vi "170131-Counter - Continuous Output.vi"(8 "error in":errorcluster, 10 "Frequency":dbl=30.0 format="%.6f") -> (0 "error out 2":errorcluster={"status"=TRUE, "code"=-200220, "source"="DAQmx Create Channel (CO-Pulse Generation-Frequency).vi:4680002<append>\n<B>Device Specified: </B>Dev1\n<B>Suggested Device(s): </B>Dev4\n\n<B>Task Name: </B>_unnamedTask<4>"})   [LabVIEW 2017]
doc: "This example demonstrates how to continuously generate digital pulses using a counter output."
uses:
  <vilib>/DAQmx/create/channels.llb/DAQmx Create Channel (CO-Pulse Generation-Frequency).vi
  <vilib>/DAQmx/configure/timing.llb/DAQmx Timing (Implicit).vi
  <vilib>/DAQmx/configure/trigger.llb/DAQmx Start Trigger (Digital Edge).vi
  Global_InitEndSync.vi
  <resource>/objmgr/daqmx.rc
  <vilib>/Utility/error.llb/DialogType.ctl
panel:
  out "Actual Duty Cycle":dbl
  out "Actual Frequency":dbl
  in  "Duty Cycle":dbl=0.5 format="%.6f"
  in  "Output Terminal":tag="/PXI1Slot2/PFI24"
  in  "Trigger Type":T1(tab)
  in  "Edge":i32(ring)=10280 items=["Rising"=10280, "Falling"=10171]
  in  "Digital Trigger Source":tag
  in  "Pause When":i32(ring)=10192 items=["High"=10192, "Low"=10214]
  in  "Pause Trigger Source":tag
  in  "Stop":bool
  in  "Counter":tag="PXI1Slot2/ctr3"
  # "Channel Settings"
  # "Trigger Settings"
  # "To configure and use a trigger you must have the necessary tab selected above."
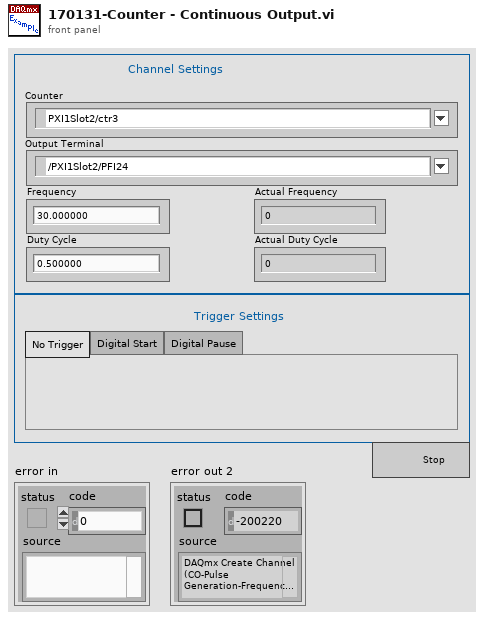
[diagram p1: front panel]
types:
  T1 = enum32{"No Trigger", "Digital Start", "Digital Pause"}
  T2 = typedef "DialogType.ctl" = u16
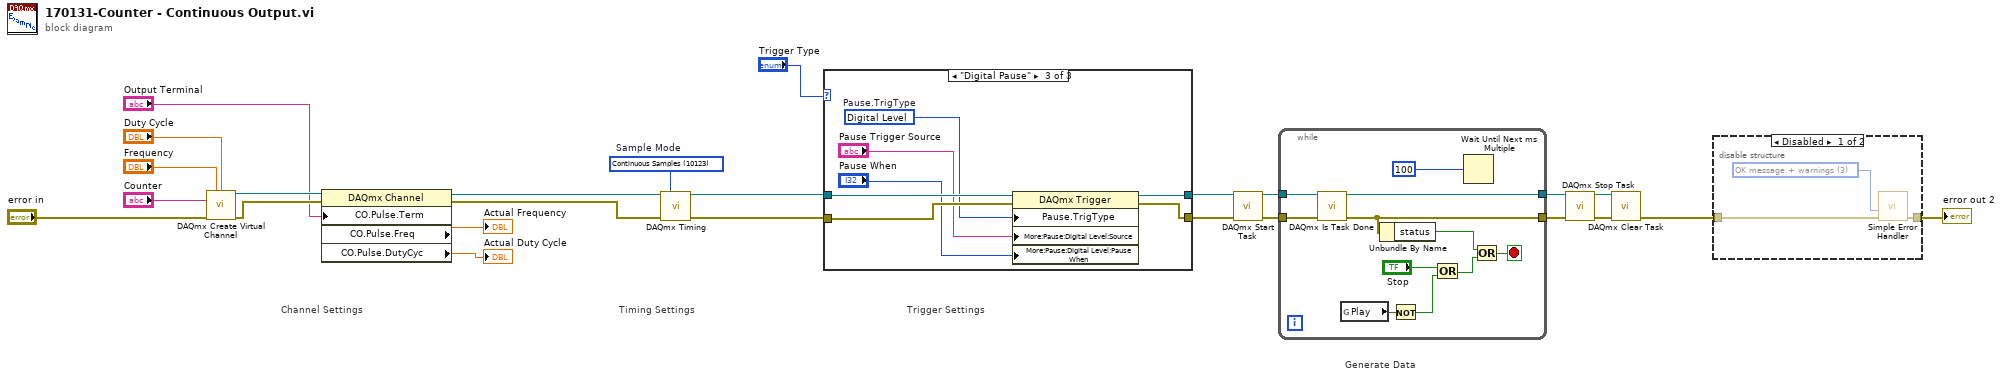
[diagram p0: block diagram]
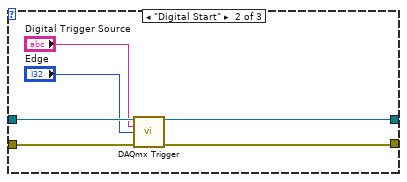
[diagram p4: hidden frame]
diagram:
  w25 = 10123 items=["Finite Samples"=10178, "Continuous Samples"=10123, "Hardware Timed Single Point"=12522]  # Sample Mode
  # "Generate Data"
  # "Trigger Settings"
  # "Timing Settings"
  # "Channel Settings"
  n1 = call-poly <vilib>:"DAQmx Create Virtual Channel.vi"("frequency"="Frequency", "duty cycle"="Duty Cycle", "counter"="Counter", "error in"="error in") -> ("task out"=w15:refnum<k21>, "error out"=w14:errorcluster)  [unwired: 10 in]
  n2 = property class="DAQmx Channel"(reference=w15, error in=w14, "CO.Pulse.Term"="Output Terminal") -> (reference out=w11:refnum<k21>, error out=w12:errorcluster, "CO.Pulse.Freq"=→"Actual Frequency":dbl, "CO.Pulse.DutyCyc"=→"Actual Duty Cycle":dbl)
  n3 = call-poly <vilib>:"DAQmx Timing.vi"("task/channels in"=w11, "sample mode"=w25, "error in"=w12) -> ("task out"=w19:refnum<k21>, "error out"=w18:errorcluster)  [unwired: 11 in]
  n4 = case shown="\"Digital Pause\"" "Trigger Type" {
    tunnel: w19 -> [w27 w33 w40]
    tunnel: w18 -> [w26 w32 w37]
    tunnel: [w27 w31 w39] -> w16
    tunnel: [w26 w30 w38] -> w17
    frame "No Trigger", Default {
    }
    frame "Digital Start" {
      n5 = call-poly <vilib>:"DAQmx Trigger.vi"("task/channels in"=w33, "source"="Digital Trigger Source", "edge"="Edge", "error in"=w32) -> ("task out"=w31:refnum<k21>, "error out"=w30:errorcluster)  [unwired: 10 in]
    }
    frame "Digital Pause" {
      w36 = 10152 items=["Analog Level"=10101, "Analog Window"=10103, "Digital Level"=10152, "Digital Pattern"=10398, "None"=10230]  # Pause.TrigType
      n6 = property class="DAQmx Trigger"(reference=w40, error in=w37, "Pause.TrigType"=w36, "More:Pause:Digital Level:Source"="Pause Trigger Source", "More:Pause:Digital Level:Pause When"="Pause When") -> (reference out=w39:refnum<k21>, error out=w38:errorcluster)
    }
  }
  n7 = call <vilib>:"DAQmx Start Task.vi"("task/channels in"=w16, "error in"=w17) -> ("task out"=w24:refnum<k21>, "error out"=w23:errorcluster)  [unwired: 12 in]
  n8 = while {
    tunnel: w24 -> [w51]
    tunnel: w23 -> [w50]
    tunnel: [w47] -> w3
    tunnel: [w48] -> w4
    stop <- w49 stop-if-true
    n9 = call <vilib>:"DAQmx Is Task Done.vi"("task/channels in"=w51, "error in"=w50) -> ("task out"=w48:refnum<k21>, "error out"=w47:errorcluster)  [unwired: 11 in, 1 out]
    n10 = global read "Global_InitEndSync.vi" "Play"() -> (w42:bool)
    n11 = Unbundle By Name(w47) -> ("status"=w46:bool)
    n12 = Not(x=w42) -> (.not. x?=w41:bool)
    n13 = Or(x="Stop", y=w41) -> (x .or. y?=w43:bool)
    n14 = Wait Until Next ms Multiple(millisecond multiple=u32 100) -> ()  [unwired: 1 out]
    n15 = Or(x=w46, y=w43) -> (x .or. y?=w49:bool)
  }
  n16 = call <vilib>:"DAQmx Stop Task.vi"("task/channels in"=w4, "error in"=w3) -> ("task out"=w6:refnum<k21>, "error out"=w5:errorcluster)  [unwired: 12 in]
  n17 = call <vilib>:"DAQmx Clear Task.vi"("task in"=w6, "error in"=w5) -> ("error out"=w22:errorcluster)  [unwired: 13 in]
  n18 = disable-structure shown="Disabled" {
    disable-tunnel: w22 -> [w54 _]
    disable-tunnel: [w52 _] -> w1
    frame Disabled {
      w53 = T2 3 items=["no dialog", "OK message", "continue or stop message", "OK message + warnings", "continue/stop + warnings"] ("type of dialog (OK msg:1)")
      n19 = call <vilib>:"Simple Error Handler.vi"("type of dialog (OK msg:1)"=w53, "error in (no error)"=w54) -> ("error out"=w52:errorcluster)  [unwired: 3 in, 4 out]
    }
    frame Enabled {
    }
  }
  "error out 2" <- w1
